vi "Configure Trace Operation.vi"(0 "VISA resource name":refnum<visa-resource-name>, 1 "Math Operation (0: Power Diff)":i32(ring) items=["Power Diff", "Power Sum", "Log Offset", "Log Diff", "Off"], 2 "Log Offset (0 dB)":dbl, 5 "Trace Operand 1 (1: Trace 1)":i32(ring)=1 items=["Trace 1"=1, "Trace 2"=2, "Trace 3"=3, "Trace 4"=4, "Trace 5"=5, "Trace 6"=6], 7 "Destination Trace (1: Trace 1)":i32(ring)=1 items=["Trace 1"=1, "Trace 2"=2, "Trace 3"=3, "Trace 4"=4, "Trace 5"=5, "Trace 6"=6], 9 "Trace Operand 2 (2: Trace 2)":i32(ring)=2 items=["Trace 1"=1, "Trace 2"=2, "Trace 3"=3, "Trace 4"=4, "Trace 5"=5, "Trace 6"=6], 11 "error in (no error)":errorcluster, 13 "Log Difference Reference (0 dBm)":dbl) -> (4 "VISA resource name out":refnum<visa-resource-name>, 15 "error out":errorcluster)   [LabVIEW 2018, in "Agilent MXA Series.lvlib"]
doc: "Configure the trace operation.\n\n<B>Note:</B>\nYou can use this VI only under Swept SA measurement type."
uses:
  Agilent MXA Series.lvlib
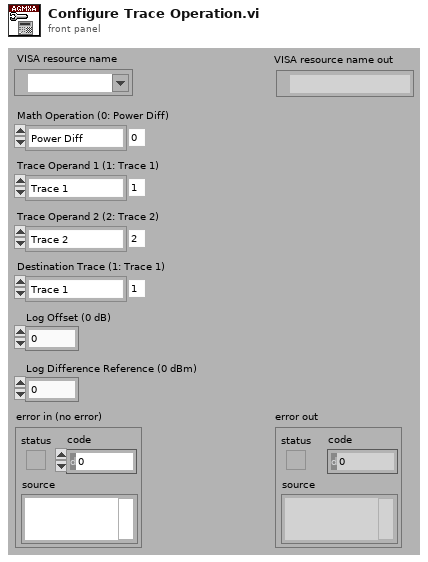
[diagram p1: front panel]
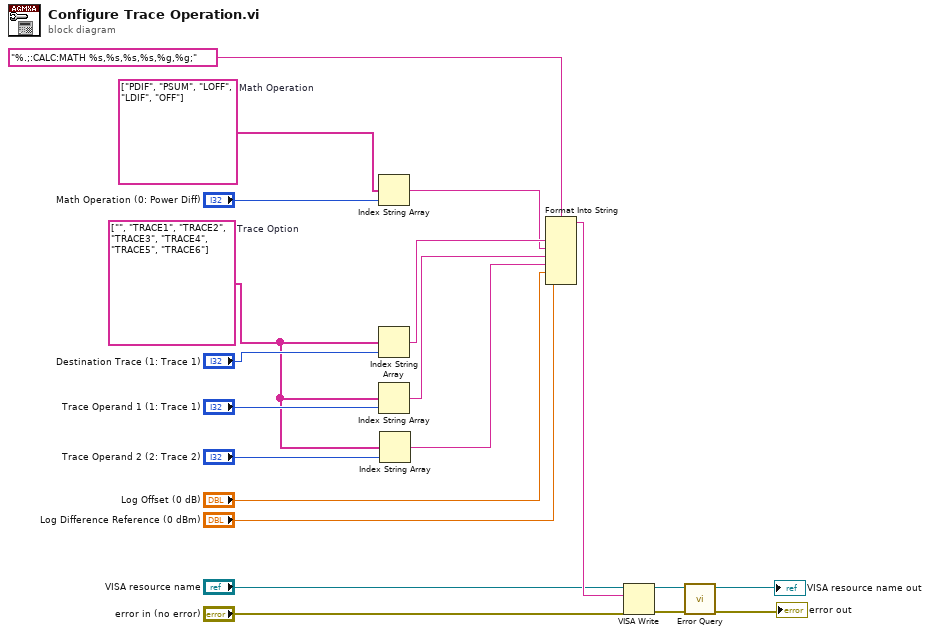
[diagram p0: block diagram]
diagram:
  w1 = string[] ["", "TRACE1", "TRACE2", "TRACE3", "TRACE4", "TRACE5", "TRACE6"]  # Trace Option
  w19 = string[] ["PDIF", "PSUM", "LOFF", "LDIF", "OFF"]  # Math Operation
  n1 = Index String Array(1:"Math Operation (0: Power Diff)", 2:w19) -> (0:w11:string)  [unwired: 1 in]
  n2 = Index String Array(1:"Destination Trace (1: Trace 1)", 2:w1) -> (0:w12:string)  [unwired: 1 in]
  n3 = Index String Array(1:"Trace Operand 1 (1: Trace 1)", 2:w1) -> (0:w15:string)  [unwired: 1 in]
  n4 = Index String Array(1:"Trace Operand 2 (2: Trace 2)", 2:w1) -> (0:w14:string)  [unwired: 1 in]
  n5 = Format Into String(format string="%.;:CALC:MATH %s,%s,%s,%s,%g,%g;", w12, w11, w15, w14, "Log Offset (0 dB)", "Log Difference Reference (0 dBm)") -> (resulting string=w8:string)  [unwired: 2 in, 1 out]
  n6 = VISA Write(VISA resource name="VISA resource name", write buffer=w8, error in (no error)="error in (no error)") -> (VISA resource name out=w5:refnum<visa-resource-name>, error out=w4:errorcluster)  [unwired: 1 out]
  n7 = call "Error Query.vi"("error in (no error)"=w4, "VISA resource name"=w5) -> ("error out"=→"error out":errorcluster, "VISA resource name out"=→"VISA resource name out":refnum<visa-resource-name>)  [unwired: 6 in, 2 out]
